vi "Size to Largest.vi"(6 "Secondary Default In":variant, 7 "Primary Default In":variant, 9 "Secondary Array In":variant[](array[variant]), 11 "Primary Array In":variant[](array[variant])) -> (1 "Secondary Array Out":variant[](array[variant]), 3 "Primary Array Out":variant[](array[variant]))   [LabVIEW 2015]
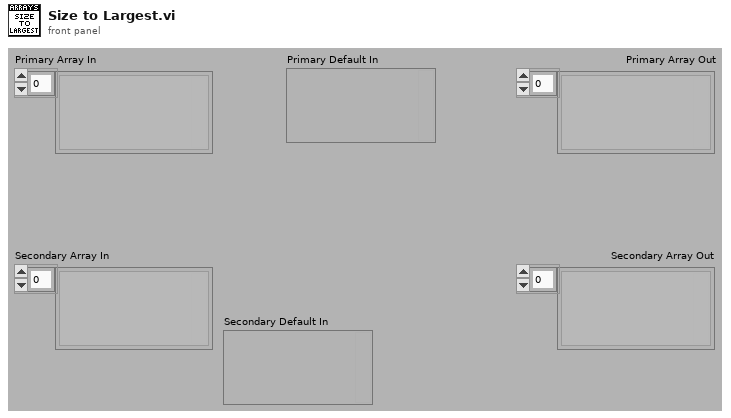
[diagram p1: front panel]
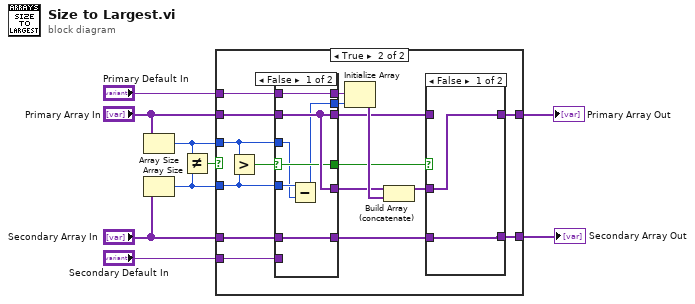
[diagram p0: block diagram]
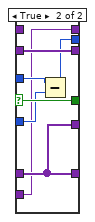
[diagram p4: hidden frame]
diagram:
  n1 = Array Size(array="Primary Array In") -> (size(s)=w2:i32)
  n2 = Array Size(array="Secondary Array In") -> (size(s)=w3:i32)
  n3 = Not Equal?(x=w2, y=w3) -> (x != y?=w1:bool)
  n4 = case shown="True" w1 {
    tunnel: "Secondary Default In" -> [_ w23]
    tunnel: "Primary Default In" -> [_ w22]
    tunnel: [w11 w20] -> w7
    tunnel: [w10 w17] -> w6
    tunnel: "Secondary Array In" -> [w10 w15]
    tunnel: w3 -> [_ w14]
    tunnel: "Primary Array In" -> [w11 w13]
    tunnel: w2 -> [_ w12]
    frame False {
    }
    frame True {
      n5 = Greater?(x=w12, y=w14) -> (0:w16:bool)
      n6 = case shown="False" w16 {
        selector: w16 -> [w37 w44]
        tunnel: [w38 w45] -> w26
        tunnel: w13 -> [w38 w46]
        tunnel: [w39 w45] -> w18
        tunnel: w15 -> [w39 w45]
        tunnel: [w38 w46] -> w19
        tunnel: [w37 w44] -> w21
        tunnel: w14 -> [w36 w42]
        tunnel: [w34 w41] -> w25
        tunnel: w12 -> [w35 w43]
        tunnel: w22 -> [w33 _]
        tunnel: [w33 w40] -> w24
        tunnel: w23 -> [_ w40]
        frame False {
          n7 = Subtract(x=w36, y=w35) -> (x-y=w34:i32)
        }
        frame True {
          n8 = Subtract(x=w43, y=w42) -> (x-y=w41:i32)
        }
      }
      n9 = Initialize Array(w24, w25) -> (w28:variant[])
      n10 = Build Array (concatenate)(w26, w28) -> (w27:variant[])
      n11 = case shown="False" w21 {
        tunnel: w27 -> [w30 w32]
        tunnel: [w29 w32] -> w17
        tunnel: w18 -> [w29 _]
        tunnel: w19 -> [_ w31]
        tunnel: [w30 w31] -> w20
        frame False {
        }
        frame True {
        }
      }
    }
  }
  "Primary Array Out" <- w7
  "Secondary Array Out" <- w6
